vi "Queue Is Nested.vi"(10 "Alias":string, 11 "Actor in":refnum<class "Actor.lvclass">) -> (2 "Queue Is Nested?":bool)   [LabVIEW 2021, in "jettl.lvlib" / "Actor.lvclass"]
uses:
  Actor.lvclass
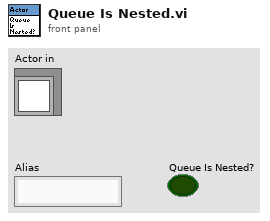
[diagram p1: front panel]
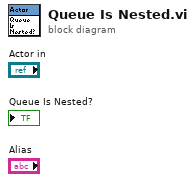
[diagram p0: block diagram]
diagram:
